vi "ErrorLog.vi"(7 "Case":enum16{"ErrorHandler", "Initialize", "Quit"}(ring), 8 "error in (no error)":errorcluster) -> (0 "error out":errorcluster)   [LabVIEW 2012, in "ErrorLog_lib.lvlib"]
uses:
  <userlib>/Utility/ErrorLog_lib.lvlib
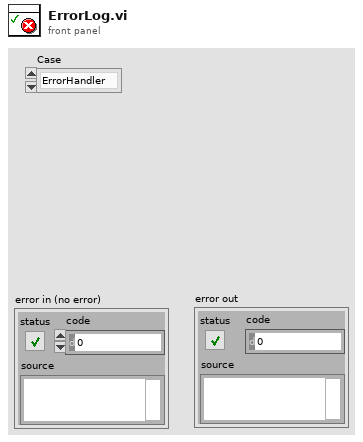
[diagram p1: front panel]
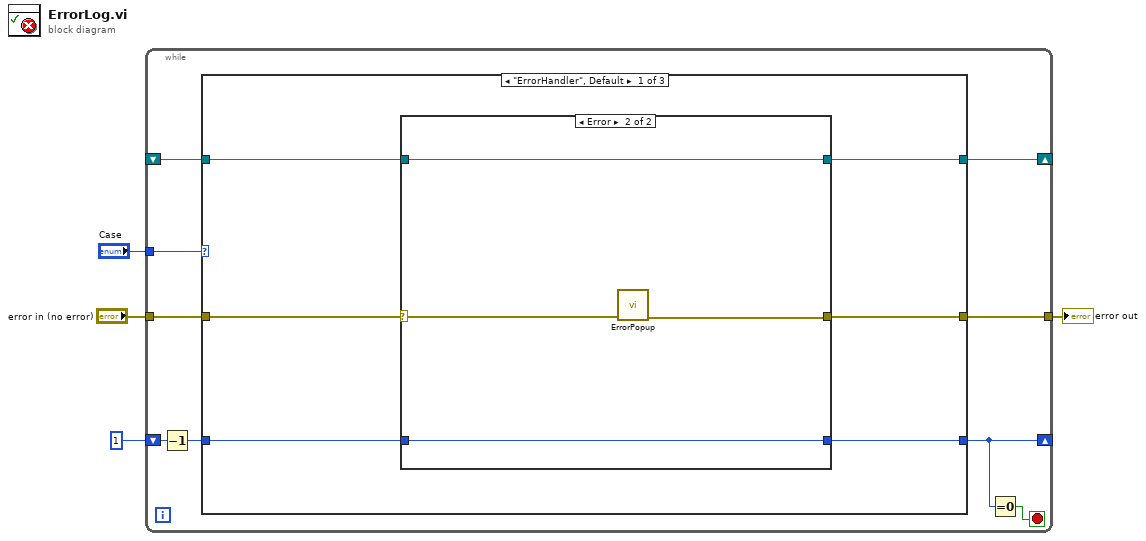
[diagram p0: block diagram]
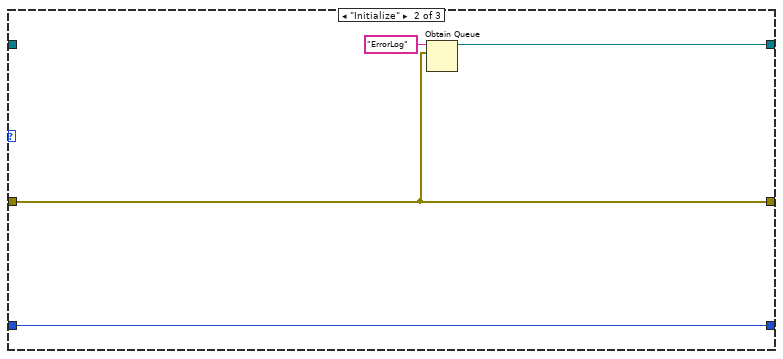
[diagram p3: hidden frame]
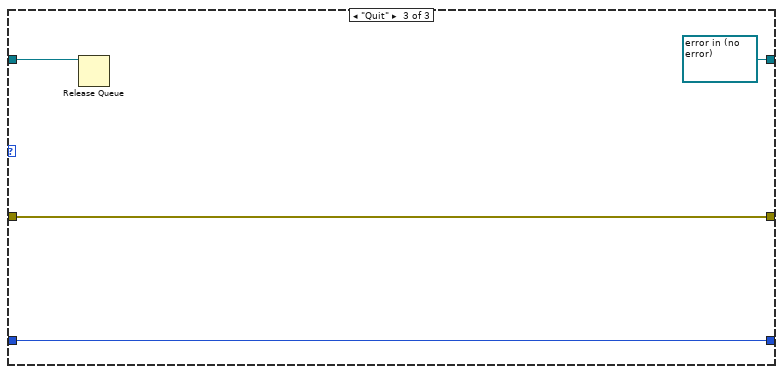
[diagram p4: hidden frame]
diagram:
  n1 = while {
    tunnel: "error in (no error)" -> [w13]
    tunnel: [w12] -> w3
    shift-right: [w5] -> _
    shift-left: 1 -> [w10]
    tunnel: "Case" -> [w11]
    shift-right: [w9] -> _
    shift-left: _ -> [w8]
    stop <- w6 stop-if-true
    n2 = Decrement(x=w10) -> (x-1=w7:i32)
    n3 = case shown="\"ErrorHandler\", Default" w11 {
      tunnel: w13 -> [w19 w27 w32]
      tunnel: [w18 w27 w32] -> w12
      tunnel: [w17 w30 w34] -> w5
      tunnel: w7 -> [w16 w30 w34]
      tunnel: [w14 w29 refnum<queue> refnum ("queue out")] -> w9
      tunnel: w8 -> [w15 _ w33]
      frame "ErrorHandler", Default {
        n4 = case shown="Error" w19 {
          selector: w19 -> [w22 w24]
          tunnel: [w22 w23] -> w18
          tunnel: [w21 w25] -> w17
          tunnel: w16 -> [w21 w25]
          tunnel: w15 -> [w20 w26]
          tunnel: [w20 w26] -> w14
          frame No Error {
          }
          frame Error {
            n5 = call <userlib>:"ErrorPopup.vi"("error in (no error)"=w24) -> ("error out"=w23:errorcluster)  [unwired: 10 in]
          }
        }
      }
      frame "Initialize" {
        n6 = Obtain Queue(name (unnamed)="ErrorLog", element data type=w27) -> (queue out=w29:refnum<queue>)  [unwired: 3 in, 2 out]
      }
      frame "Quit" {
        n7 = Release Queue(queue=w33) -> ()  [unwired: 2 in, 3 out]
      }
    }
    n8 = Equal To 0?(x=w5) -> (x = 0?=w6:bool)
  }
  "error out" <- w3
